vi "ReadToNull.vi"(8 "error in (no error)":errorcluster, 11 "VISA resource name":refnum<visa-resource-name>) -> (0 "error out":errorcluster, 2 "read buffer":string, 3 "VISA resource name out":refnum<visa-resource-name>)   [LabVIEW 2015, in "Ion Motion Roboclaw.lvlib"]
uses:
  <instrlib>/Ion Motion Roboclaw/Ion Motion Roboclaw.lvlib
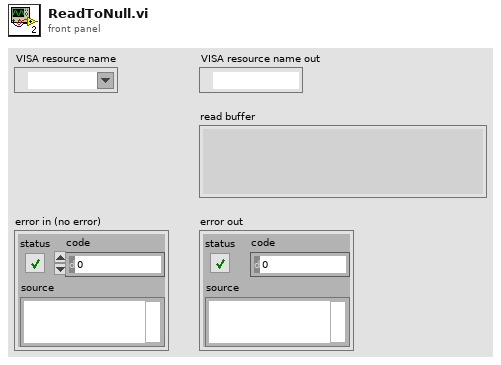
[diagram p1: front panel]
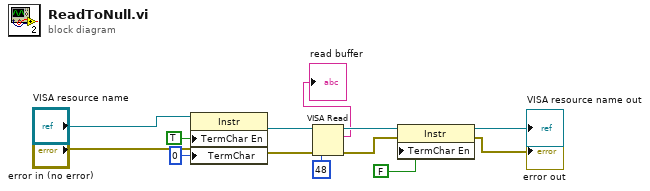
[diagram p0: block diagram]
diagram:
  n1 = property class="Instr"(reference="VISA resource name", "TermChar En"=TRUE ("Message Based Settings:Termination Character Enable"), "TermChar"=u8 0 ("Message Based Settings:Termination Character")) -> (reference out=w3:refnum<visa-resource-name>)  [unwired: 1 in, 1 out]
  n2 = VISA Read(VISA resource name=w3, byte count=u32 48, error in (no error)="error in (no error)") -> (VISA resource name out=w12:refnum<visa-resource-name>, read buffer=→"read buffer":string, error out=w9:errorcluster)  [unwired: 1 out]
  n3 = property class="Instr"(reference=w12, error in=w9, "TermChar En"=FALSE ("Message Based Settings:Termination Character Enable")) -> (reference out=→"VISA resource name out":refnum<visa-resource-name>, error out=→"error out":errorcluster)
